vi "ExcelReadConfigFile.vi"(0 "NomProjet":string, 2 "error in (no error)":errorcluster) -> (3 "ConfigurationTotale":T1, 6 "error out":errorcluster)   [LabVIEW 2017]
uses:
  DefDeType/ConfigTotale.ctl
  DefDeType/VoltageChannels.ctl
  DefDeType/WBridgeChannels.ctl
  DefDeType/Configuration.ctl
  DefDeType/WhichPath.ctl
panel:
  out "EndString":string
  out "StartString":string
  in  "Excel._Worksheet 2":refnum<k7>
  in  "Array":string[][](array[string])
  in  "Excel._Worksheet":refnum<k7>
  in  "Excel._Application":refnum<k7>
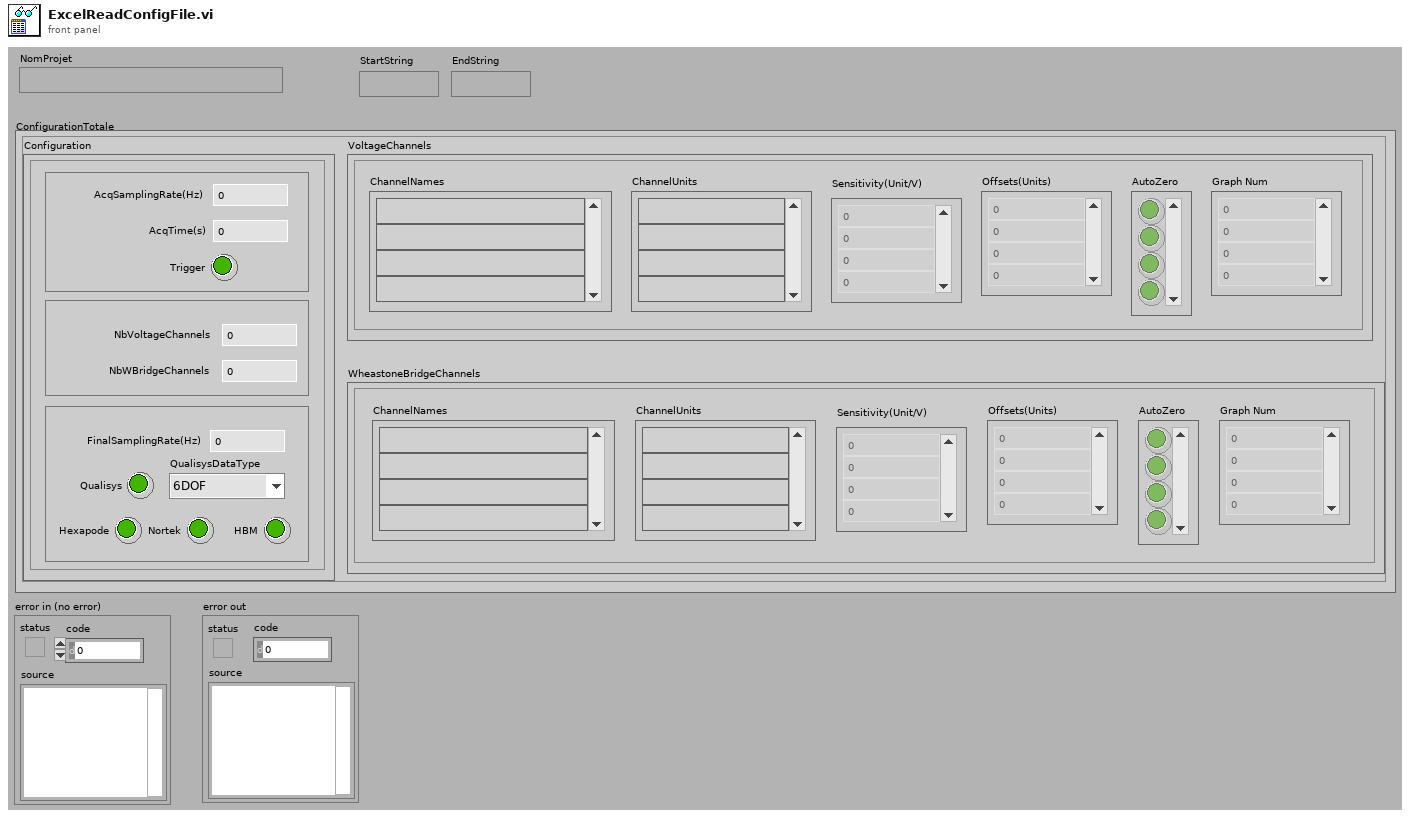
[diagram p1: front panel]
types:
  T1 = typedef "ConfigTotale.ctl" = cluster{"VoltageChannels":T2, "WheastoneBridgeChannels":T3, "Configuration":T4}
  T2 = typedef "VoltageChannels.ctl" = cluster{"ChannelNames":string[], "Sensitivity(Unit/V)":dbl[], "AutoZero":bool[], "ChannelUnits":string[], "Offsets(Units)":dbl[], "Graph Num":u8[]}
  T3 = typedef "WBridgeChannels.ctl" = cluster{"ChannelNames":string[], "Sensitivity(Unit/V)":dbl[], "AutoZero":bool[], "ChannelUnits":string[], "Offsets(Units)":dbl[], "Graph Num":u8[]}
  T4 = typedef "Configuration.ctl" = cluster{"AcqSamplingRate(Hz)":u32, "AcqTime(s)":u32, "Trigger":bool, "NbVoltageChannels":u32, "NbWBridgeChannels":u32, "Qualisys":bool, "Hexapode":bool, "FinalSamplingRate(Hz)":u32, "QualisysDataType":enum16{"6DOF", "3DTracking", "6DOF + 3D"}, "Nortek":bool, "HBM":bool}
  T5 = typedef "WhichPath.ctl" = enum16{"DossierProjet", "Config", "Meas", "MeasPCI", "MeasCRIO1", "MeasCRIO2", "MeasQualisys", "MeasHBM", "MeasTDMS", "Fig", "Res"}
  T6 = cluster{"Start Row":i32, "Start Column":i32, "End Row":i32, "End Column":i32}[]
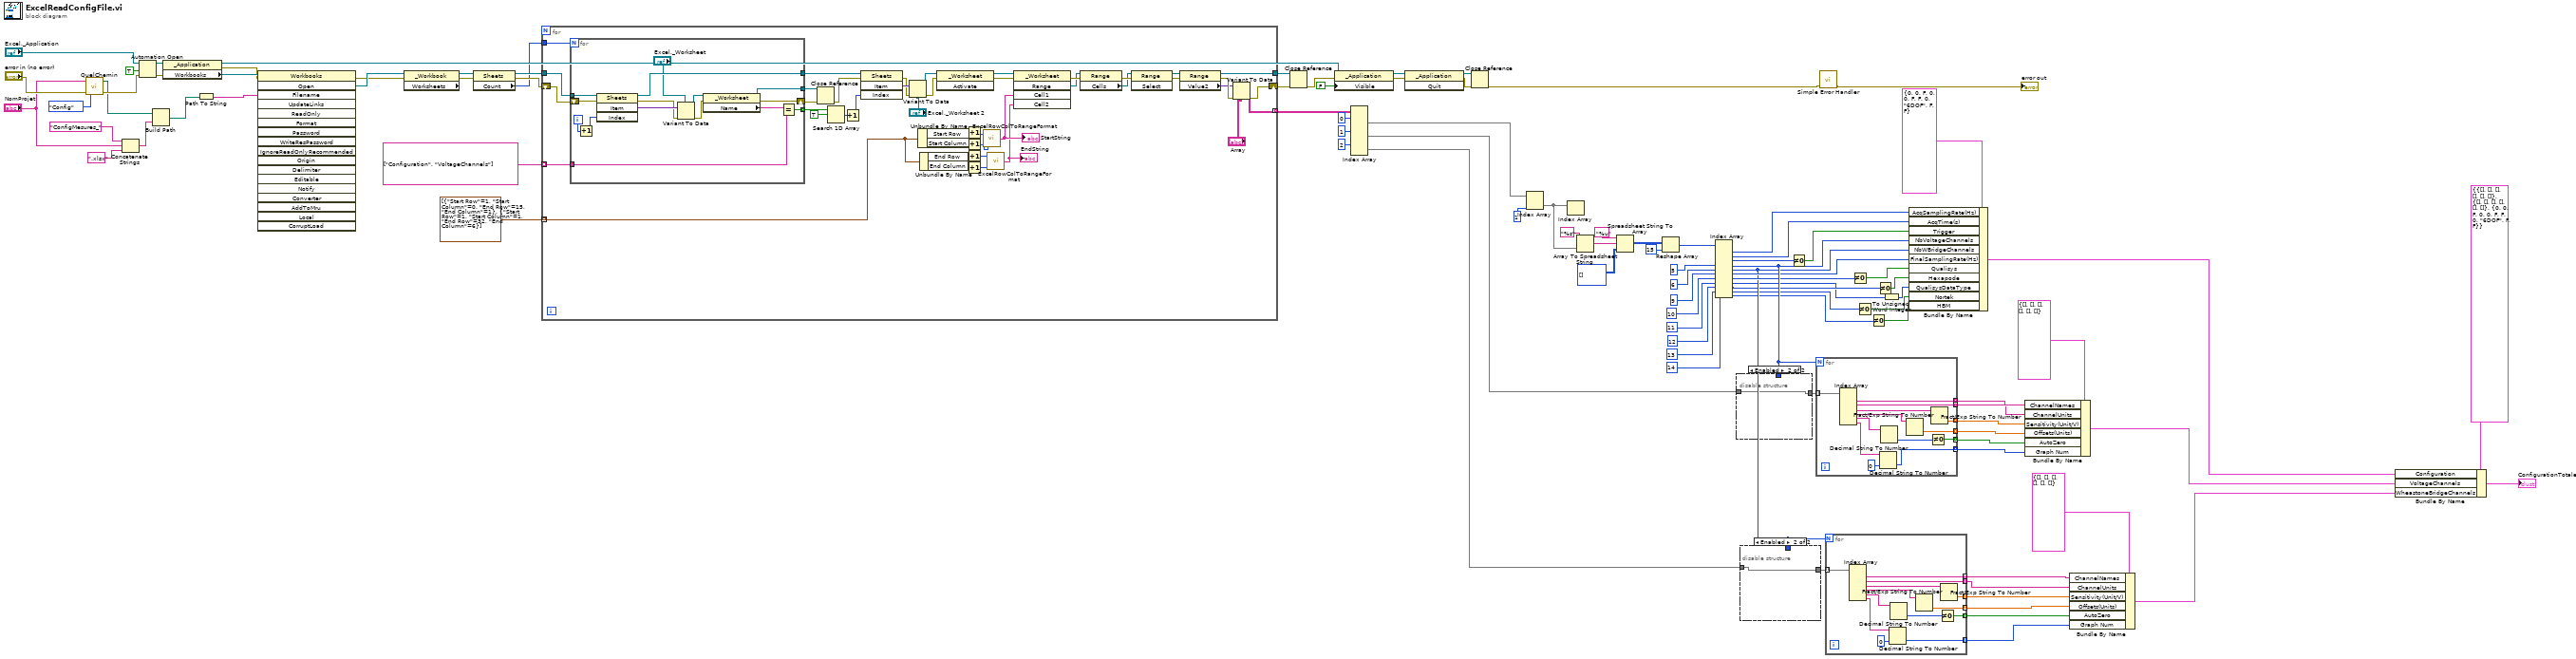
[diagram p0: block diagram]
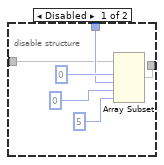
[diagram p2: hidden frame]
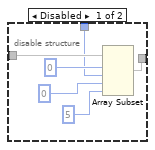
[diagram p3: hidden frame]
diagram:
  n1 = call "QuelChemin.vi"("Entrée d'erreur"="error in (no error)", "WhichPath?"=WhichPath."Config", "NomProjet"="NomProjet") -> ("Sortie d'erreur"=w51:errorcluster, "SurDisqueLocal"=w48:path)  [unwired: 1 out]
  n2 = Concatenate Strings("ConfigMesures_" ("nom ou chemin relatif"), "NomProjet", ".xlsx" ("nom ou chemin relatif")) -> (w53:string)
  n3 = Automation Open(error in (no error)=w51, Automation Refnum="Excel._Application", 9:TRUE ("ouvrir une nouvelle instance (faux)")) -> (Automation Refnum=w98:refnum<k7>, error out=w97:errorcluster)  [unwired: 1 in]
  n4 = Build Path(base path=w48, name or relative path=w53) -> (appended path=w77:path)
  n5 = property class="_Application"(reference=w98, error in=w97) -> (reference out=w91:refnum<k7>, error out=w94:errorcluster, "Workbooks"=w95:refnum<k7>)
  n6 = Path To String(path=w77) -> (string=w78:string)
  n7 = invoke class="Workbooks" method="Open"(reference=w95, error in=w94, "Filename"=w78) -> (error out=w92:errorcluster, "Open"=w93:refnum<k7>)  [unwired: 15 in, 16 out]
  n8 = property class="_Workbook"(reference=w93, error in=w92) -> (error out=w84:errorcluster, "Worksheets"=w85:refnum<k7>)  [unwired: 1 out]
  n9 = property class="Sheets"(reference=w85, error in=w84) -> (reference out=w83:refnum<k7>, error out=w82:errorcluster, "Count"=w81:i32)
  n10 = for {
    tunnel: [w134] -> w88
    tunnel: w83 -> [w131]
    tunnel: w81 -> [w123]
    tunnel: [w102] -> w74 mode=indexing
    shift-right: [w133] -> w87
    shift-left: w82 -> [w127]
    tunnel: string[] ["Configuration", "VoltageChannels"] -> [w101] mode=indexing
    tunnel: T6 [{"Start Row"=1, "Start Column"=0, "End Row"=15, "End Column"=1}, {"Start Row"=1, "Start Column"=1, "End Row"=32, "End Column"=6}] -> [w100] mode=indexing
    n11 = for {
      N: w123 -> [_]
      tunnel: w131 -> [w156]
      shift-right: [w146] -> w122
      shift-left: w127 -> [w155]
      tunnel: [w147] -> w124 mode=indexing
      tunnel: [w145] -> w125
      tunnel: [w144] -> w120
      tunnel: w101 -> [w142]
      i -> [w153]
      n12 = Increment(x=w153) -> (x+1=w154:i32)
      n13 = invoke class="Sheets" method="Item"(reference=w156, error in=w155, "Index"=w154) -> (reference out=w145:refnum<k7>, error out=w151:errorcluster, "Item"=w152:variant)  [unwired: 1 in, 1 out]
      n14 = Variant To Data(error in=w151, type="Excel._Worksheet", Variant=w152) -> (data=w149:refnum<k7>, error out=w150:errorcluster)
      n15 = property class="_Worksheet"(reference=w149, error in=w150) -> (reference out=w144:refnum<k7>, error out=w146:errorcluster, "Name"=w148:string)
      n16 = Equal?(x=w148, y=w142) -> (x = y?=w147:bool)
    }
    n17 = Close Reference(reference=w120, error in (no error)=w122) -> (error out=w121:errorcluster)
    n18 = Search 1D Array(1D array=w124, element=TRUE) -> (index of element=w129:i32)  [unwired: 1 in]
    n19 = Increment(x=w129) -> (x+1=w128:i32)
    n20 = invoke class="Sheets" method="Item"(reference=w125, error in=w121, "Index"=w128) -> (error out=w140:errorcluster, "Item"=w141:variant)  [unwired: 1 in, 2 out]
    n21 = Variant To Data(error in=w140, type="Excel._Worksheet 2", Variant=w141) -> (data=w119:refnum<k7>, error out=w139:errorcluster)
    n22 = Unbundle By Name(w100) -> ("Start Row"=w114:i32, "Start Column"=w113:i32)
    n23 = Unbundle By Name(w100) -> ("End Row"=w112:i32, "End Column"=w111:i32)
    n24 = invoke class="_Worksheet" method="Activate"(reference=w119, error in=w139) -> (reference out=w116:refnum<k7>, error out=w115:errorcluster)  [unwired: 1 in, 1 out]
    n25 = Increment(x=w114) -> (x+1=w107:i32)
    n26 = Increment(x=w113) -> (x+1=w106:i32)
    n27 = Increment(x=w112) -> (x+1=w105:i32)
    n28 = Increment(x=w111) -> (x+1=w104:i32)
    n29 = call "ExcelRowColToRangeFormat.vi"("Column"=w106, "Row"=w107) -> ("Output String"=w108:string)
    "StartString" <- w108
    n30 = call "ExcelRowColToRangeFormat.vi"("Column"=w104, "Row"=w105) -> ("Output String"=w103:string)
    "EndString" <- w103
    n31 = invoke class="_Worksheet" method="Range"(reference=w116, error in=w115, "Cell1"=w108, "Cell2"=w103) -> (error out=w110:errorcluster, "Range"=w109:refnum<k7>)  [unwired: 1 in, 3 out]
    n32 = property class="Range"(reference=w109, error in=w110) -> (error out=w138:errorcluster, "Cells"=w118:refnum<k7>)  [unwired: 1 out]
    n33 = invoke class="Range" method="Select"(reference=w118, error in=w138) -> (reference out=w137:refnum<k7>, error out=w136:errorcluster)  [unwired: 1 in, 1 out]
    n34 = property class="Range"(reference=w137, error in=w136) -> (reference out=w134:refnum<k7>, error out=w135:errorcluster, "Value2"=w132:variant)
    n35 = Variant To Data(error in=w135, type="Array", Variant=w132) -> (data=w102:string[][], error out=w133:errorcluster)
  }
  n36 = Close Reference(reference=w88, error in (no error)=w87) -> (error out=w86:errorcluster)
  n37 = property class="_Application"(reference=w91, error in=w86, "Visible"=FALSE) -> (reference out=w89:refnum<k7>, error out=w90:errorcluster)
  n38 = Index Array(array=w74, index (dim 0) #1=0 ("indice (page)"), index (dim 0) #2=1 ("indice (page)"), index (dim 0) #3=2 ("indice (page)")) -> (element #1=w62:string[][], element #2=w60:string[][], element #3=w30:string[][])  [unwired: 6 in]
  n39 = invoke class="_Application" method="Quit"(reference=w89, error in=w90) -> (reference out=w80:refnum<k7>, error out=w79:errorcluster)  [unwired: 1 in, 1 out]
  n40 = Close Reference(reference=w80, error in (no error)=w79) -> (error out=w58:errorcluster)
  n41 = Index Array(array=w62, index (col)=1 ("indice désactivé (col)")) -> (element=w66:string[])  [unwired: 1 in]
  n42 = Index Array(array=w66) -> ()  [unwired: 1 in, 1 out]
  n43 = Array To Spreadsheet String(array=w66, 3:"%s" ("format string")) -> (spreadsheet string=w69:string)  [unwired: 1 in]
  n44 = Spreadsheet String To Array(format string="%u", spreadsheet string=w69, array type (2D Dbl)=u32[][] [] ("type de tableau (2D de dbl)")) -> (array=w65:u32[][])  [unwired: 1 in]
  n45 = Reshape Array(w65, 15 ("taille de la dimension")) -> (w64:u32[])
  n46 = Index Array(array=w64, index #4=5 ("taille de la dimension"), index #5=6 ("taille de la dimension"), index #6=9 ("taille de la dimension"), index #7=10 ("taille de la dimension"), index #8=11 ("taille de la dimension"), index #9=12 ("taille de la dimension"), index #10=13 ("taille de la dimension"), index #11=14 ("taille de la dimension")) -> (element #1=w44:u32, element #2=w43:u32, element #3=w42:u32, element #4=w37:u32, element #5=w31:u32, element #6=w33:u32, element #7=w36:u32, element #8=w10:u32, element #9=w11:u32, element #10=w7:u32, element #11=w2:u32)  [unwired: 3 in]
  n47 = disable-structure shown="Enabled" {
    disable-tunnel: [w162 w163] -> w61
    disable-tunnel: w60 -> [w161 w163]
    disable-tunnel: w37 -> [w157 _]
    frame Disabled {
      n48 = Array Subset(array=w161, index (row)=0 ("indice"), length (row)=w157, index (col)=0 ("indice"), length (col)=5 ("longueur")) -> (w162:string[][])
    }
    frame Enabled {
    }
  }
  n49 = disable-structure shown="Enabled" {
    disable-tunnel: [w166 w170] -> w32
    disable-tunnel: w31 -> [w165 _]
    disable-tunnel: w30 -> [w164 w170]
    frame Disabled {
      n50 = Array Subset(array=w164, index (row)=0 ("indice"), length (row)=w165, index (col)=0 ("indice"), length (col)=5 ("longueur")) -> (w166:string[][])
    }
    frame Enabled {
    }
  }
  n51 = Not Equal To 0?(x=w42) -> (x != 0?=w41:bool)
  n52 = for {
    N: w37 -> [_]
    tunnel: w61 -> [w183] mode=indexing
    tunnel: [w182] -> w28 mode=indexing
    tunnel: [w181] -> w27 mode=indexing
    tunnel: [w179] -> w26 mode=indexing
    tunnel: [w177] -> w25 mode=indexing
    tunnel: [w174] -> w24 mode=indexing
    tunnel: [w171] -> w5 mode=indexing
    n53 = Index Array(array=w183) -> (element #1=w182:string, element #2=w181:string, element #3=w180:string, element #4=w178:string, element #5=w176:string, element #6=w173:string)  [unwired: 6 in]
    n54 = Decimal String To Number(string=w173, default (0L)=u8 0 ("default (0 I32)")) -> (number=w171:u8)  [unwired: 1 in, 1 out]
    n55 = Decimal String To Number(string=w176) -> (number=w175:i32)  [unwired: 2 in, 1 out]
    n56 = Fract/Exp String To Number(string=w178) -> (number=w177:dbl)  [unwired: 3 in, 1 out]
    n57 = Not Equal To 0?(x=w175) -> (x != 0?=w174:bool)
    n58 = Fract/Exp String To Number(string=w180) -> (number=w179:dbl)  [unwired: 3 in, 1 out]
  }
  n59 = call <vilib>:"Simple Error Handler.vi"("error in (no error)"=w58) -> ("error out"=→"error out":errorcluster)  [unwired: 4 in, 4 out]
  n60 = for {
    N: w31 -> [_]
    tunnel: w32 -> [w196] mode=indexing
    tunnel: [w195] -> w22 mode=indexing
    tunnel: [w194] -> w21 mode=indexing
    tunnel: [w192] -> w20 mode=indexing
    tunnel: [w190] -> w19 mode=indexing
    tunnel: [w187] -> w18 mode=indexing
    tunnel: [w184] -> w4 mode=indexing
    n61 = Index Array(array=w196) -> (element #1=w195:string, element #2=w194:string, element #3=w193:string, element #4=w191:string, element #5=w189:string, element #6=w185:string)  [unwired: 6 in]
    n62 = Decimal String To Number(string=w185, default (0L)=u8 0 ("default (0 I32)")) -> (number=w184:u8)  [unwired: 1 in, 1 out]
    n63 = Decimal String To Number(string=w189) -> (number=w188:i32)  [unwired: 2 in, 1 out]
    n64 = Fract/Exp String To Number(string=w191) -> (number=w190:dbl)  [unwired: 3 in, 1 out]
    n65 = Not Equal To 0?(x=w188) -> (x != 0?=w187:bool)
    n66 = Fract/Exp String To Number(string=w193) -> (number=w192:dbl)  [unwired: 3 in, 1 out]
  }
  n67 = Not Equal To 0?(x=w36) -> (x != 0?=w34:bool)
  n68 = Not Equal To 0?(x=w7) -> (x != 0?=w6:bool)
  n69 = Not Equal To 0?(x=w2) -> (x != 0?=w1:bool)
  n70 = Not Equal To 0?(x=w11) -> (x != 0?=w35:bool)
  n71 = To Unsigned Word Integer(number=w10) -> (unsigned 16bit integer=w9:u16)
  n72 = Bundle By Name(cluster=T4 {"AcqSamplingRate(Hz)"=0, "AcqTime(s)"=0, "Trigger"=FALSE, "NbVoltageChannels"=0, "NbWBridgeChannels"=0, "Qualisys"=FALSE, "Hexapode"=FALSE, "FinalSamplingRate(Hz)"=0, "QualisysDataType"=enum."6DOF", "Nortek"=FALSE, "HBM"=FALSE} ("Configuration"), "AcqSamplingRate(Hz)"=w44, "AcqTime(s)"=w43, "Trigger"=w41, "NbVoltageChannels"=w37, "NbWBridgeChannels"=w31, "FinalSamplingRate(Hz)"=w33, "Qualisys"=w34, "Hexapode"=w35, "QualisysDataType"=w9, "Nortek"=w6, "HBM"=w1) -> (w16:T4)
  n73 = Bundle By Name(cluster=T2 {"ChannelNames"=[], "Sensitivity(Unit/V)"=[], "AutoZero"=[], "ChannelUnits"=[], "Offsets(Units)"=[], "Graph Num"=[]} ("VoltageChannels"), "ChannelNames"=w28, "ChannelUnits"=w27, "Sensitivity(Unit/V)"=w26, "Offsets(Units)"=w25, "AutoZero"=w24, "Graph Num"=w5) -> (w15:T2)
  n74 = Bundle By Name(cluster=T3 {"ChannelNames"=[], "Sensitivity(Unit/V)"=[], "AutoZero"=[], "ChannelUnits"=[], "Offsets(Units)"=[], "Graph Num"=[]} ("WheastoneBridgeChannels"), "ChannelNames"=w22, "ChannelUnits"=w21, "Sensitivity(Unit/V)"=w20, "Offsets(Units)"=w19, "AutoZero"=w18, "Graph Num"=w4) -> (w14:T3)
  n75 = Bundle By Name(cluster=T1 {"VoltageChannels"={"ChannelNames"=[], "Sensitivity(Unit/V)"=[], "AutoZero"=[], "ChannelUnits"=[], "Offsets(Units)"=[], "Graph Num"=[]}, "WheastoneBridgeChannels"={"ChannelNames"=[], "Sensitivity(Unit/V)"=[], "AutoZero"=[], "ChannelUnits"=[], "Offsets(Units)"=[], "Graph Num"=[]}, "Configuration"={"AcqSamplingRate(Hz)"=0, "AcqTime(s)"=0, "Trigger"=FALSE, "NbVoltageChannels"=0, "NbWBridgeChannels"=0, "Qualisys"=FALSE, "Hexapode"=FALSE, "FinalSamplingRate(Hz)"=0, "QualisysDataType"=enum."6DOF", "Nortek"=FALSE, "HBM"=FALSE}} ("ConfigTotale"), "Configuration"=w16, "VoltageChannels"=w15, "WheastoneBridgeChannels"=w14) -> (→"ConfigurationTotale":T1)
